vi "Set Drive Outputs.vi"(8 "Rear Right":dbl, 9 "Rear Left":dbl, 10 "Front Right":dbl, 11 "Front Left":dbl) -> ()   [LabVIEW 2012]
uses:
  Globals/Jaguar Commands.vi
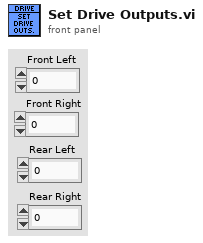
[diagram p1: front panel]
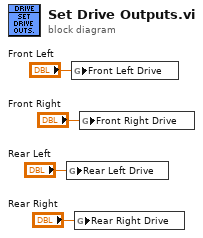
[diagram p0: block diagram]
diagram:
  n1 = global write "Jaguar Commands.vi" "Rear Left Drive"("Rear Left") -> ()
  n2 = global write "Jaguar Commands.vi" "Front Left Drive"("Front Left") -> ()
  n3 = global write "Jaguar Commands.vi" "Rear Right Drive"("Rear Right") -> ()
  n4 = global write "Jaguar Commands.vi" "Front Right Drive"("Front Right") -> ()
